vi "PathPlanner_Path_BezierFromWaypointsJSON.vi"(11 "JSON string":string) -> (0 "Error":bool, 3 "Bezier":T2[](array[typedef]) {"Y" format="%14.3f"; "X" format="%14.3f"}, 4 "value":T1(array[cluster]))   [LabVIEW 2019, in "PathPlanner.lvlib"]
doc: "Parse bezier points from a JSON string formated as waypoint.\n\nInputs: \n - JSON String - string - JSON containing waypoint to parse and convert to bezier point array\n\nOutputs:\n - Bezier - array of translation2s - List of bezier points\n - error - boolean - TRUE if an error occured.\n - value - array of cluster - bezier points -- for debugging"
uses:
  PathPlanner.lvlib
  <vilib>/Rock Robotics/WPI/ThirdParty/JAS_Junk/TrajLib/TypeDef/TRANSLATION2D.ctl
  <vilib>/Rock Robotics/WPI/ThirdParty/JAS_Junk/TrajLib/Trajectory_Library.lvlib
panel:
  in  "waypoints":T1(array[cluster])
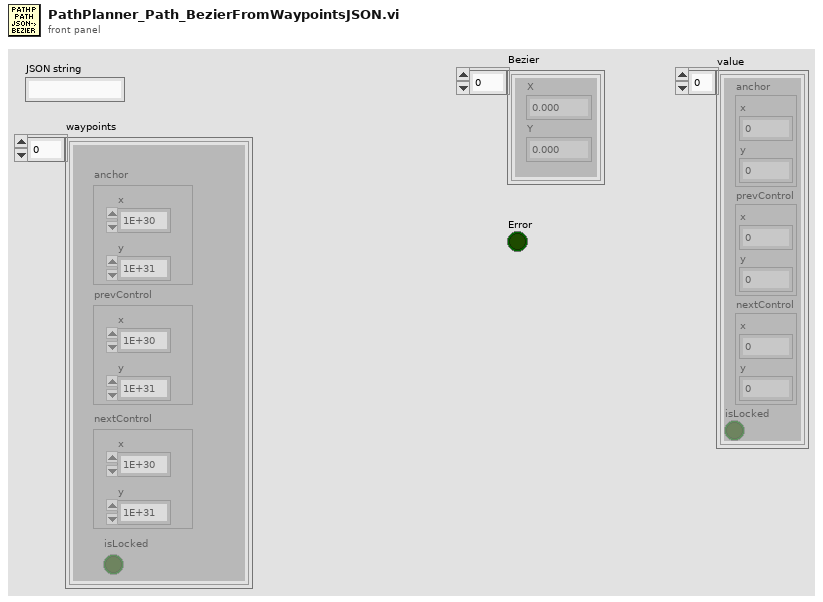
[diagram p1: front panel]
types:
  T1 = cluster{"anchor":cluster{"x":dbl, "y":dbl}, "prevControl":cluster{"x":dbl, "y":dbl}, "nextControl":cluster{"x":dbl, "y":dbl}, "isLocked":bool}[]
  T2 = typedef "Trajectory_Library.lvlib/TRANSLATION2D.ctl" = cluster{"X":dbl, "Y":dbl}
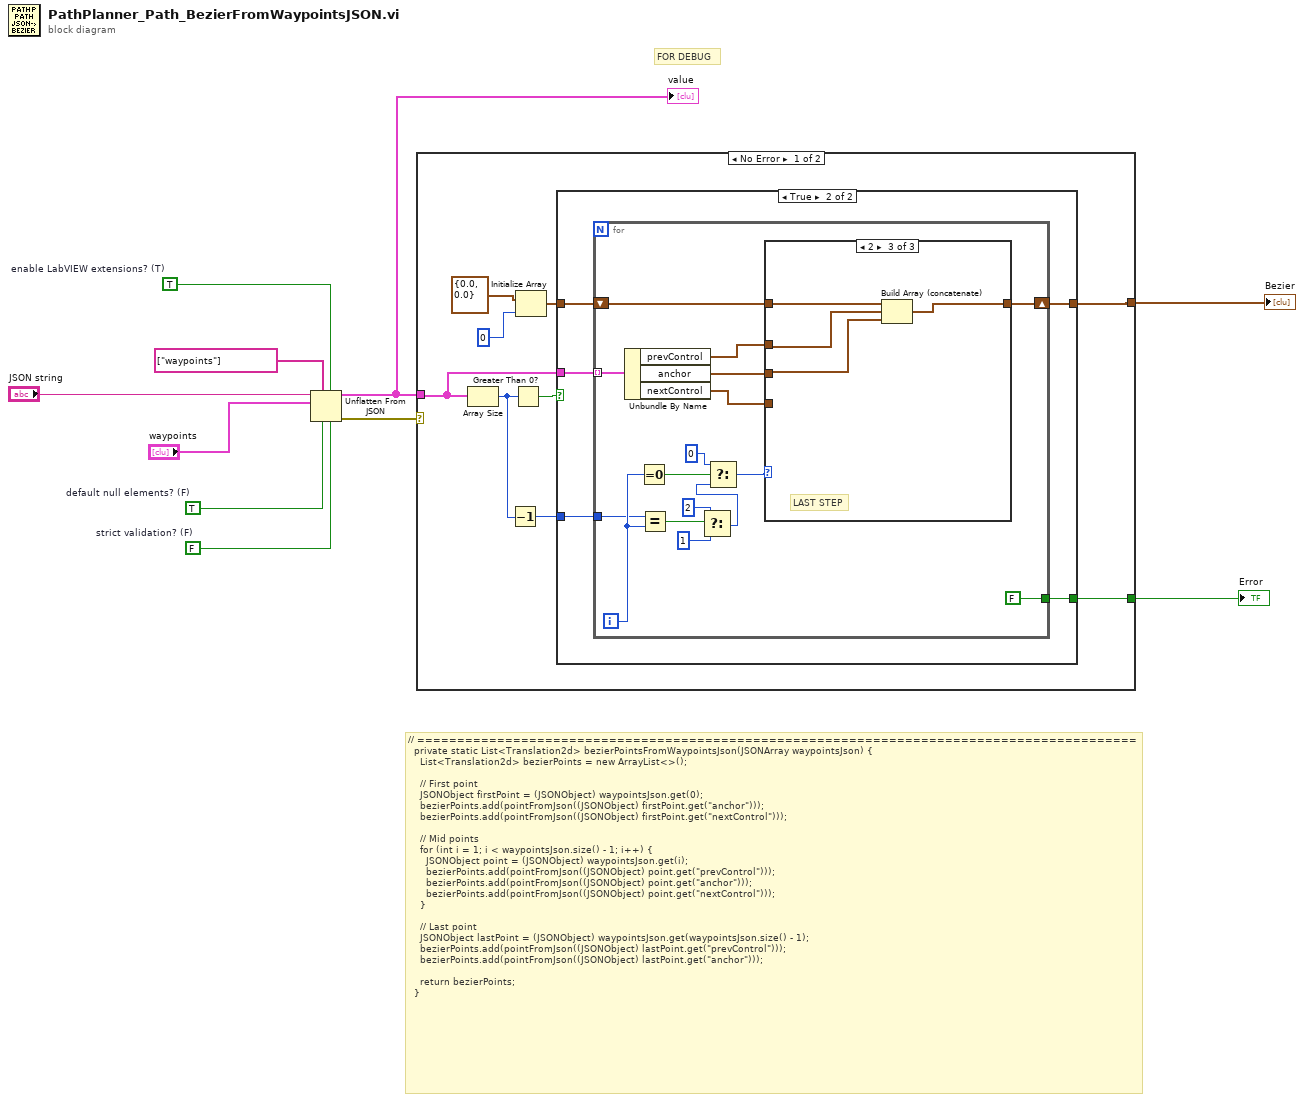
[diagram p0: block diagram]
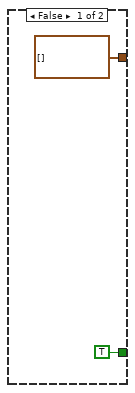
[diagram p2: hidden frame]
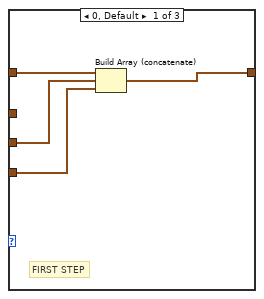
[diagram p3: hidden frame]
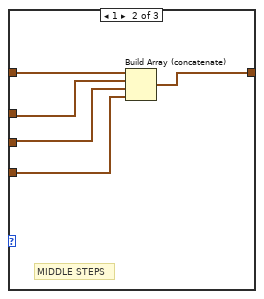
[diagram p4: hidden frame]
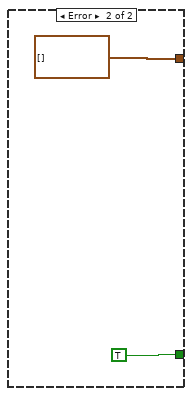
[diagram p5: hidden frame]
diagram:
  w5 = TRUE  # default null elements? (F)
  w6 = FALSE  # strict validation? (F)
  w7 = TRUE  # enable LabVIEW extensions? (T)
  # "FOR DEBUG"
  # "// ==========================================================================================\n  private static List<Translation2d> bezierPointsFromWaypointsJson(JSONArray waypointsJson) {\n    List<Translation2d> bezierPoints = new ArrayList<>();\n\n    // First point\n    JSONObject firstPoint = (JSONObject) waypointsJson.get(0);\n    bezierPoints.add(pointFromJson((JSONObject) firstPoint.get(\"anchor\")));\n    bezierPoints.add(pointFromJson((JSONObject) firstPoint.get(\"nextControl\")));\n\n    // Mid points\n    for (int i = 1; i < waypointsJson.size() - 1; i++) {\n      JSONObject point = (JSONObject) waypointsJson.get(i);\n      bezierPoints.add(pointFromJson((JSONObject) point.get(\"prevControl\")));\n      bezierPoints.add(pointFromJson((JSONObject) point.get(\"anchor\")));\n      bezierPoints.add(pointFromJson((JSONObject) point.get(\"nextControl\")));\n    }\n\n    // Last point\n    JSONObject lastPoint = (JSONObject) waypointsJson.get(waypointsJson.size() - 1);\n    bezierPoints.add(pointFromJson((JSONObject) lastPoint.get(\"prevControl\")));\n    bezierPoints.add(pointFromJson((JSONObject) lastPoint.get(\"anchor\")));\n\n    return bezierPoints;\n  }"
  n1 = Unflatten From JSON(path=string[] ["waypoints"], enable LabVIEW extensions? (T)=w7, JSON string="JSON string", type and defaults="waypoints", default null elements? (F)=w5, strict validation? (F)=w6) -> (value=w1:T1, error out=w8:errorcluster)  [unwired: 1 in]
  "value" <- w1
  n2 = case shown="No Error" w8 {
    tunnel: w1 -> [w13 _]
    tunnel: [w11 TRUE] -> w3
    tunnel: [w12 T2[] [] ("Bezier")] -> w2
    frame No Error {
      n3 = Array Size(array=w13) -> (size(s)=w18:i32)
      n4 = Decrement(x=w18) -> (x-1=w17:i32)
      n5 = Greater Than 0?(x=w18) -> (x > 0?=w19:bool)
      n6 = Initialize Array(T2 {"X"=0.0, "Y"=0.0} ("Bezier"), 0 ("dimension size")) -> (w14:T2[])
      n7 = case shown="True" w19 {
        tunnel: w17 -> [_ w26]
        tunnel: w14 -> [_ w25]
        tunnel: w13 -> [_ w24]
        tunnel: [T2[] [] w23] -> w12
        tunnel: [TRUE w22] -> w11
        frame False {
        }
        frame True {
          n8 = for {
            tunnel: w26 -> [w41]
            shift-right: [w28] -> w23
            shift-left: w25 -> [w32]
            tunnel: w24 -> [w33] mode=indexing
            tunnel: [FALSE] -> w22
            i -> [w42]
            n9 = Unbundle By Name(w33) -> ("prevControl"=w31:cluster{"x":dbl, "y":dbl}, "anchor"=w30:cluster{"x":dbl, "y":dbl}, "nextControl"=w29:cluster{"x":dbl, "y":dbl})
            n10 = Equal To 0?(x=w42) -> (x = 0?=w40:bool)
            n11 = Equal?(x=w41, y=w42) -> (x = y?=w38:bool)
            n12 = Select(t=2, s=w38, f=1) -> (s? t:f=w35:i32)
            n13 = Select(t=0, s=w40, f=w35) -> (s? t:f=w34:i32)
            n14 = case shown="2" w34 {
              tunnel: w32 -> [w46 w51 w55]
              tunnel: w31 -> [_ w50 w54]
              tunnel: w30 -> [w45 w49 w53]
              tunnel: w29 -> [w44 w48 _]
              tunnel: [w43 w47 w52] -> w28
              frame 0, Default {
                # "FIRST STEP"
                n15 = Build Array (concatenate)(w46, w45, w44) -> (w43:T2[])
              }
              frame 1 {
                # "MIDDLE STEPS"
                n16 = Build Array (concatenate)(w51, w50, w49, w48) -> (w47:T2[])
              }
              frame 2 {
                # "LAST STEP"
                n17 = Build Array (concatenate)(w55, w54, w53) -> (w52:T2[])
              }
            }
          }
        }
      }
    }
    frame Error {
    }
  }
  "Bezier" <- w2
  "Error" <- w3
